vi "DN4_2Darray1DDigitalWfm.vi"(1 "data":u8[][](array[numeric])) -> (0 "1D Wfm":digitalwaveform[](array[waveform]))   [LabVIEW 2020]
uses:
  <vilib>/Waveform/DTblOps.llb/DTbl Boolean Array to Digital.vi
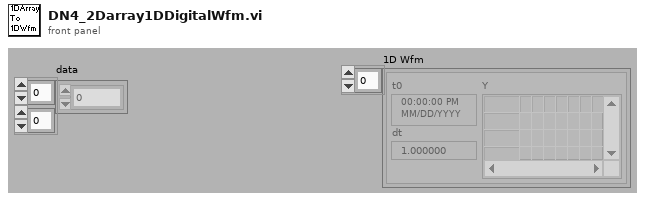
[diagram p1: front panel]
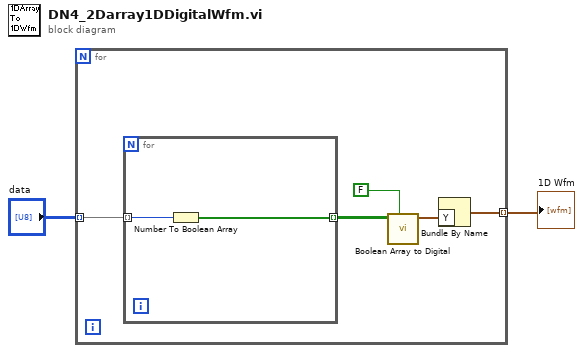
[diagram p0: block diagram]
diagram:
  n1 = for {
    tunnel: "data" -> [w7] mode=indexing
    tunnel: [w3] -> w1 mode=indexing
    n2 = for {
      tunnel: w7 -> [w9] mode=indexing
      tunnel: [w8] -> w6 mode=indexing
      n3 = Number To Boolean Array(number=w9) -> (Boolean array=w8:bool[])
    }
    n4 = call-poly <vilib>:"Boolean Array to Digital.vi"("compress data (F)"=FALSE ("compress data (T)"), "boolean array"=w6) -> ("digital data"=w4:digitaldata)  [unwired: 3 in, 6 out]
    n5 = Bundle By Name("Y"=w4) -> (w3:digitalwaveform)  [unwired: 1 out]
  }
  "1D Wfm" <- w1
